vi "CopyImageToRawMemoryARGB.vi"(8 "error in (no error)":errorcluster, 10 "Destination":T1, 11 "ARGB Image Source":refnum<data-value>) -> (0 "error out":errorcluster, 3 "Destination (Duplcate)":T1)   [LabVIEW 2020, in "g_ar_toolkit.image.lvlib"]
uses:
  g_ar_toolkit.image.lvlib
  Raw Memory Information.ctl
  Raw Memory Information Dimension.ctl
  g_ar_toolkit.common/Module Path.vi
  <vilib>/Utility/error.llb/Error Cluster From Error Code.vi
  01eda17f-9221-4e43-bf47-cf9d986167a3.vi
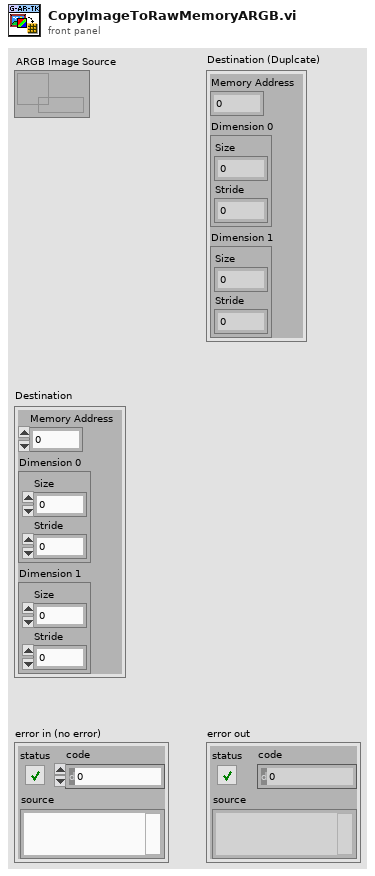
[diagram p1: front panel]
types:
  T1 = typedef "g_ar_toolkit.image.lvlib/Raw Memory Information.ctl" = cluster{"Memory Address":u64, "Dimension 0":T2, "Dimension 1":T2}
  T2 = typedef "g_ar_toolkit.image.lvlib/Raw Memory Information Dimension.ctl" = cluster{"Size":u16, "Stride":u32}
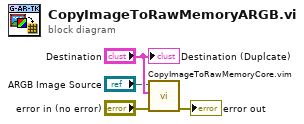
[diagram p0: block diagram]
diagram:
  n1 = call "CopyImageToRawMemoryCore.vim"("error in (no error)"="error in (no error)", "Destination"="Destination", "Src"="ARGB Image Source") -> ("error out"=→"error out":errorcluster)  [unwired: 8 in]
  "Destination (Duplcate)" <- "Destination"
